vi "二维码识别2.vi"() -> ()   [LabVIEW 2018]
uses:
  <vilib>/userdefined/High Color/IMAQdx.ctl
  <vilib>/vision/driver/NI_Vision_Acquisition_Software.lvlib
  <vilib>/vision/NI_Vision_Development_Module.lvlib
panel:
  in  "停止":bool
  out "Data":string
  out "Image":T1(plugin-control)
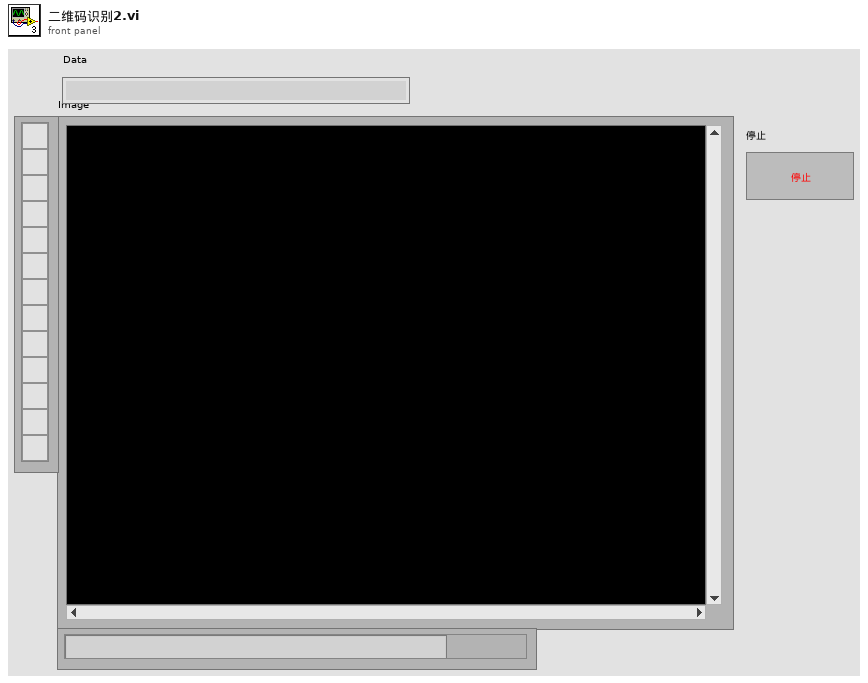
[diagram p1: front panel]
types:
  T1 = typedef "IMAQ Image.ctl" = refnum<image>
  T2 = typedef "IMAQdx.ctl" = refnum<k21>
  T3 = cluster{"Data":string, "Special Char 1":string, "Special Char 2":string, "Checksum(s)":string, "Barcode Type":u32, "Confidence Level":sgl, "Bounding Box":cluster{"x":sgl, "y":sgl}[]}[]
  T4 = cluster{"Data":string, "Special Char 1":string, "Special Char 2":string, "Checksum(s)":string, "Barcode Type":u32, "Confidence Level":sgl, "Bounding Box":cluster{"x":sgl, "y":sgl}[]}
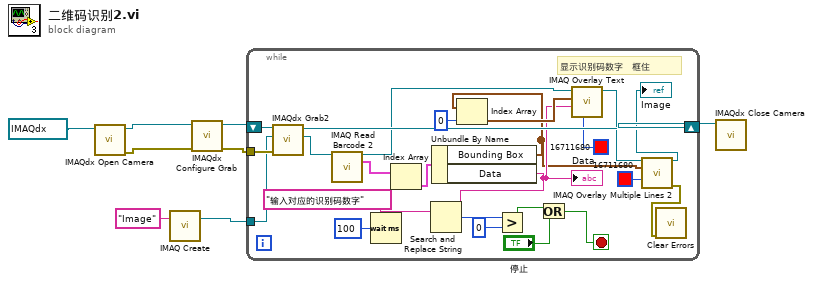
[diagram p0: block diagram]
diagram:
  n1 = call <vilib>:"IMAQdx Open Camera.vi"("Session In"=T2 "cam0") -> ("error out"=w6:errorcluster, "Session Out"=w8:T2)  [unwired: 9 in]
  n2 = call "IMAQ Create"("Image Name"="Image") -> ("New Image"=w2:T1)  [unwired: 4 in, 1 out]
  n3 = call <vilib>:"IMAQdx Configure Grab.vi"("error in"=w6, "Session In"=w8) -> ("error out"=w5:errorcluster, "Session Out"=w7:T2)  [unwired: 8 in]
  n4 = while {
    tunnel: w5 -> [w31]
    shift-right: [w30] -> w4
    shift-left: w7 -> [w32]
    tunnel: w2 -> [w28]
    stop <- w14 stop-if-true
    # "显示识别码数字   框住"
    n5 = call <vilib>:"IMAQdx Grab2.vi"("error in"=w31, "Image In"=w28, "Session In"=w32) -> ("Image Out"=w27:T1, "Session Out"=w30:T2)  [unwired: 5 in, 2 out]
    n6 = call "IMAQ Read Barcode 2"("Image"=w27) -> ("Image (duplicate)"=w21:T1, "Barcodes"=w26:T3)  [unwired: 10 in, 3 out]
    n7 = Wait (ms)(milliseconds to wait=u32 100 ("等待时间（毫秒）")) -> ()  [unwired: 1 out]
    n8 = Index Array(array=w26) -> (element=w25:T4)  [unwired: 1 in]
    n9 = Unbundle By Name(w25) -> ("Bounding Box"=w12:cluster{"x":sgl, "y":sgl}[], "Data"=w19:string)
    "Data" <- w19
    n10 = Search and Replace String(input string=w19, search string="输入对应的识别码数字" ("搜索字符串")) -> (number of replacements=w18:i32)  [unwired: 6 in, 3 out]
    n11 = Index Array(array=w12, index=0 ("索引")) -> (element=w22:cluster{"x":sgl, "y":sgl})
    n12 = Greater?(x=w18, y=0) -> (0:w16:bool)
    n13 = Or(x=w16, y="停止") -> (x .or. y?=w14:bool)
    n14 = call "IMAQ Overlay Text"("Text Color (black)"=u32 16711680, "String"=w19, "Origin"=w22, "Image"=w21) -> ("Image Out"=w13:T1)  [unwired: 6 in, 1 out]
    n15 = call "IMAQ Overlay Multiple Lines 2"("Image"=w13, "Line End Points"=w12, "Color"=u32 16711680) -> ("Image Out"=→"Image":T1, "error out"=w10:errorcluster)  [unwired: 11 in]
    n16 = call <vilib>:"Clear Errors.vi"("error in (no error)"=w10) -> ()  [unwired: 5 in, 2 out]
  }
  n17 = call <vilib>:"IMAQdx Close Camera.vi"("Session In"=w4) -> ()  [unwired: 10 in, 1 out]
